vi "RD_StepMotor_WP.vi"(8 "Step resolution":u16(ring) items=["Full step", "Half step", "1/4 step", "1/8 step", "1/16 step", "1/32 step"], 9 "Direction":bool, 10 "Time between steps (ms)":i32=1, 11 "Steps":i64=1) -> ()   [LabVIEW 2014]
doc: "André Romero - 2020\nandretec@ifsc.usp.br"
panel:
  out "Decimal number":u32
  # "DRV8825 Stepper Motor"
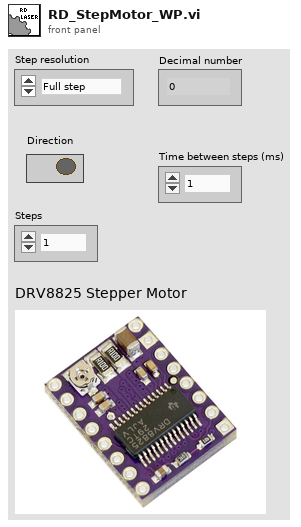
[diagram p1: front panel]
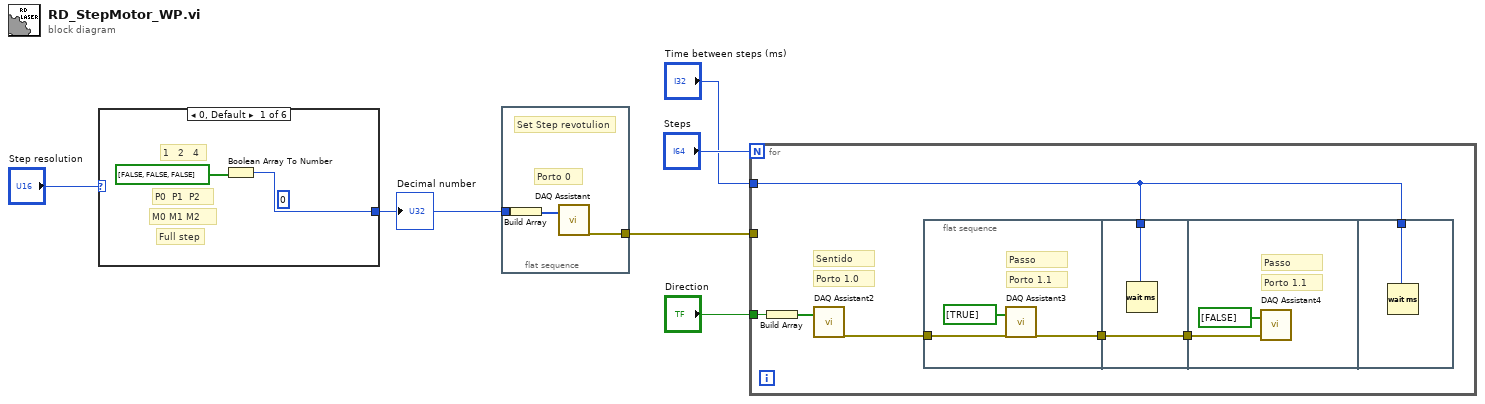
[diagram p0: block diagram]
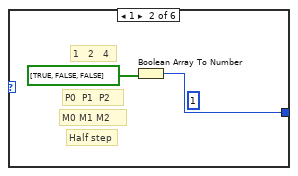
[diagram p2: hidden frame]
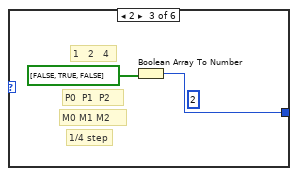
[diagram p3: hidden frame]
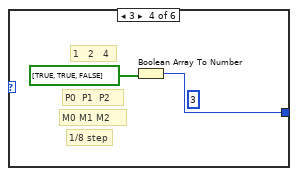
[diagram p4: hidden frame]
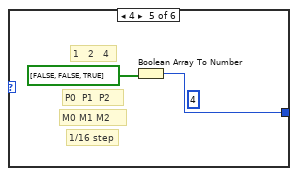
[diagram p5: hidden frame]
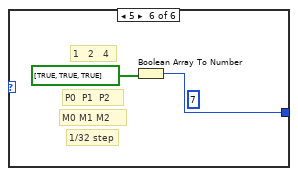
[diagram p6: hidden frame]
diagram:
  n1 = case shown="0, Default" "Step resolution" {
    tunnel: [w7 w9 w11 w13 w15 w17] -> w6
    frame 0, Default {
      (unwired) 0
      # "Full step"
      # "M0 M1 M2"
      # "P0  P1  P2"
      # "1   2   4"
      n2 = Boolean Array To Number(Boolean array=bool[] [FALSE, FALSE, FALSE]) -> (number=w7:u32)
    }
    frame 1 {
      (unwired) 1
      # "Half step"
      # "M0 M1 M2"
      # "P0  P1  P2"
      # "1   2   4"
      n3 = Boolean Array To Number(Boolean array=bool[] [TRUE, FALSE, FALSE]) -> (number=w9:u32)
    }
    frame 2 {
      (unwired) 2
      # "1/4 step"
      # "M0 M1 M2"
      # "P0  P1  P2"
      # "1   2   4"
      n4 = Boolean Array To Number(Boolean array=bool[] [FALSE, TRUE, FALSE]) -> (number=w11:u32)
    }
    frame 3 {
      (unwired) 3
      # "1/8 step"
      # "M0 M1 M2"
      # "P0  P1  P2"
      # "1   2   4"
      n5 = Boolean Array To Number(Boolean array=bool[] [TRUE, TRUE, FALSE]) -> (number=w13:u32)
    }
    frame 4 {
      (unwired) 4
      # "1/16 step"
      # "M0 M1 M2"
      # "P0  P1  P2"
      # "1   2   4"
      n6 = Boolean Array To Number(Boolean array=bool[] [FALSE, FALSE, TRUE]) -> (number=w15:u32)
    }
    frame 5 {
      (unwired) 7
      # "1/32 step"
      # "M0 M1 M2"
      # "P0  P1  P2"
      # "1   2   4"
      n7 = Boolean Array To Number(Boolean array=bool[] [TRUE, TRUE, TRUE]) -> (number=w17:u32)
    }
  }
  "Decimal number" <- w6
  n8 = flat-sequence {
    tunnel: w6 -> [w20]
    tunnel: [w19] -> w3
    frame #0 {
      # "Porto 0"
      # "Set Step revotulion"
      n9 = Build Array(w20) -> (w21:u32[])
      n10 = call "DAQ Assistant"("data"=w21) -> ("error out"=w19:errorcluster)  [unwired: 17 in, 1 out]
    }
  }
  n11 = for {
    N: "Steps" -> [_]
    tunnel: w3 -> [_]
    tunnel: "Direction" -> [w26]
    tunnel: "Time between steps (ms)" -> [w24]
    # "Sentido"
    # "Porto 1.0"
    n12 = Build Array(w26) -> (w27:bool[])
    n13 = call "DAQ Assistant2"("data"=w27) -> ("error out"=w25:errorcluster)  [unwired: 17 in, 1 out]
    n14 = flat-sequence {
      tunnel: w25 -> [w30]
      tunnel: [w28] -> w23
      tunnel: w24 -> [w32]
      tunnel: w23 -> [w31]
      tunnel: [w31] -> w22
      tunnel: w22 -> [w33]
      tunnel: w24 -> [w35]
      frame #0 {
        # "Passo"
        # "Porto 1.1"
        n15 = call "DAQ Assistant3"("data"=bool[] [TRUE], "error in"=w30) -> ("error out"=w28:errorcluster)  [unwired: 16 in, 1 out]
      }
      frame #1 {
        n16 = Wait (ms)(milliseconds to wait=w32) -> ()  [unwired: 1 out]
      }
      frame #2 {
        # "Passo"
        # "Porto 1.1"
        n17 = call "DAQ Assistant4"("data"=bool[] [FALSE], "error in"=w33) -> ()  [unwired: 16 in, 2 out]
      }
      frame #3 {
        n18 = Wait (ms)(milliseconds to wait=w35) -> ()  [unwired: 1 out]
      }
    }
  }
